vi "Alpha3.4.vi"() -> ()   [LabVIEW 2011]
uses:
  <vilib>/vision/NI_Vision_Development_Module.lvlib
panel:
  out "Image Enhanced":T1(plugin-control)
  in  "Kernel (Filters)":sgl[][](array[numeric])=array171x171[29241 elements]
  in  "Gray Morphology Operation":T2(ring)
  in  "Gamma":sgl(slide)=2.14 scale=0.0..10.0
  in  "Contrast":u8(slide)=60 scale=0.0..255.0
  in  "Brightness":u8(slide)=118 scale=0.0..255.0
  in  "Basic Morphology Operatoin":T3(ring)
  out "Contour Line":T1(plugin-control)
  in  "Threshold":cluster{u8, u8}(slide)={0, 6} scale=0.0..256.0
  in  "Stop":bool
  in  "Browse":bool
  out "Original Image":T1(plugin-control)
  out "Path to Image":path
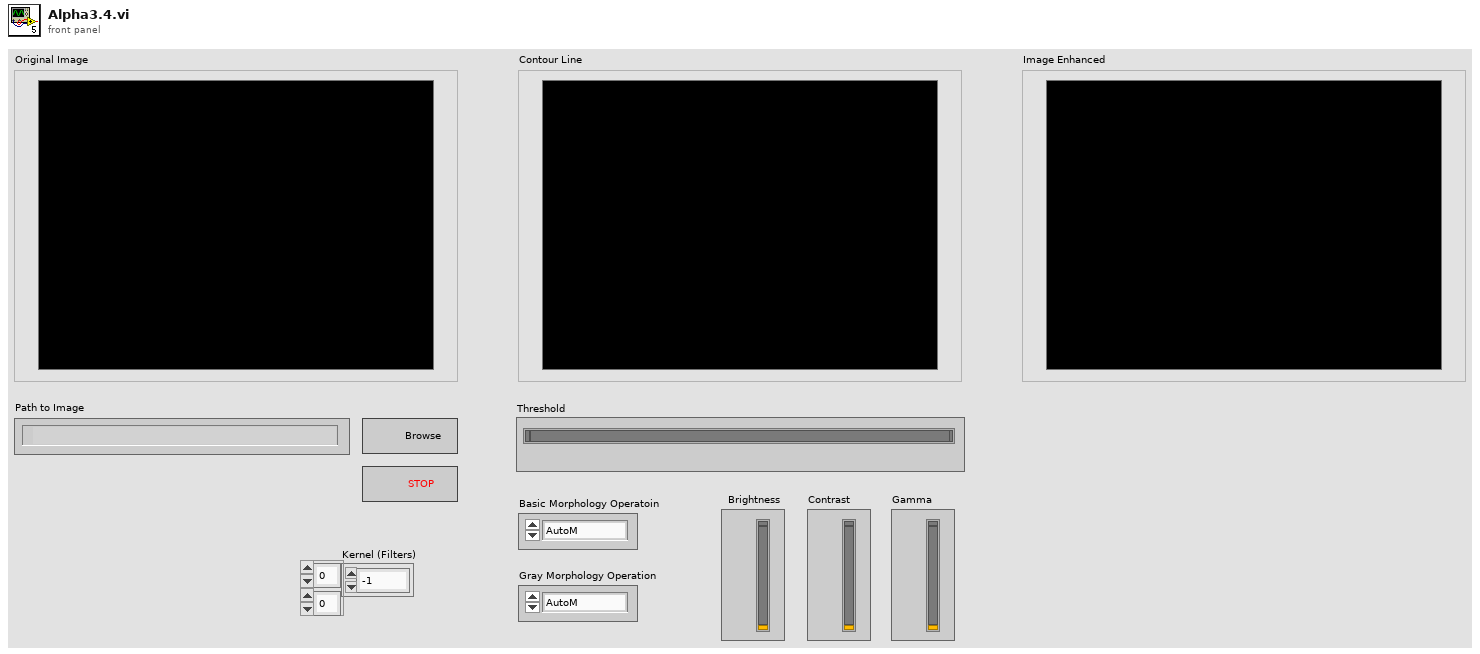
[diagram p1: front panel]
types:
  T1 = typedef "IMAQ Image.ctl" = refnum<image>
  T2 = enum16{"AutoM", "Close", "Dilate", "Erode", "Gradient", "Gradient in", "Gradient out", "HitMiss", "Open", "PClose", "POpen", "Thick", "Thin"}
  T3 = enum16{"AutoM", "Close", "Dilate", "Erode", "Gradient", "Gradient out", "Gradient in", "Hit miss", "Open", "PClose", "POpen", "Thick", "Thin"}
  T4 = typedef "Image Type" = u32
  T5 = cluster{"Brightness":u8, "Contrast":u8, "Gamma":sgl}
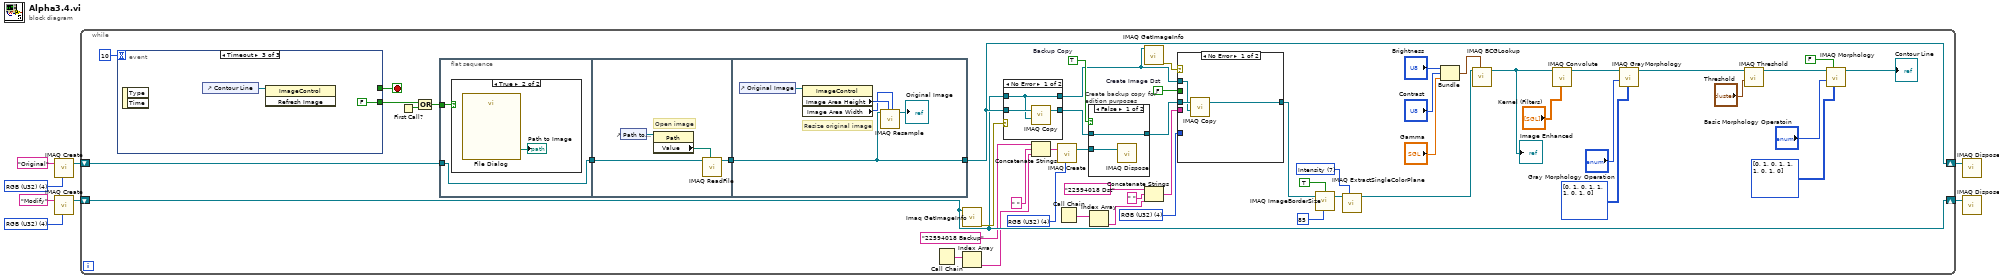
[diagram p0: block diagram]
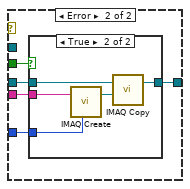
[diagram p2: hidden frame]
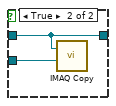
[diagram p4: hidden frame]
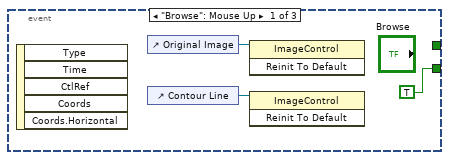
[diagram p7: hidden frame]
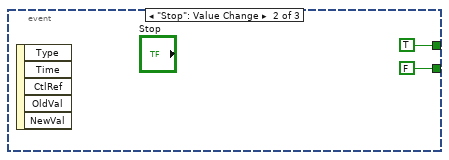
[diagram p8: hidden frame]
diagram:
  w1 = T4 4 items=["Grayscale (U8)", "Grayscale (I16)", "Grayscale (SGL)", "Complex (CSG)", "RGB (U32)", "HSL (U32)", "RGB (U64)", "Grayscale (U16)"] ("Image Type")
  w4 = T4 4 items=["Grayscale (U8)", "Grayscale (I16)", "Grayscale (SGL)", "Complex (CSG)", "RGB (U32)", "HSL (U32)", "RGB (U64)", "Grayscale (U16)"] ("Image Type")
  n1 = call "IMAQ Create"("Image Name"="Original", "Image Type"=w4) -> ("New Image"=w7:T1)  [unwired: 3 in, 1 out]
  n2 = call "IMAQ Create"("Image Name"="Modify", "Image Type"=w1) -> ("New Image"=w5:T1)  [unwired: 3 in, 1 out]
  n3 = while {
    shift-right: [w57] -> w3
    shift-left: w7 -> [w52]
    shift-right: [w56] -> w2
    shift-left: w5 -> [w56]
    stop <- w58 stop-if-true
    w38 = 7 items=["Red", "Green", "Blue", "Hue", "Saturation", "Luminance", "Value", "Intensity"] ("Color Plane")
    w34 = T4 4 items=["Grayscale (U8)", "Grayscale (I16)", "Grayscale (SGL)", "Complex (CSG)", "RGB (U32)", "HSL (U32)", "RGB (U64)", "Grayscale (U16)"] ("Image Dst Type")
    w33 = T4 4 items=["Grayscale (U8)", "Grayscale (I16)", "Grayscale (SGL)", "Complex (CSG)", "RGB (U32)", "HSL (U32)", "RGB (U64)", "Grayscale (U16)"] ("Image Type")
    w18 = TRUE  # Backup Copy
    w21 = FALSE  # Create Image Dst
    n4 = event shown="[2] Timeout" {
      selector: _ -> [_ _ _]
      dyn-events: _ -> [_ _ _]
      timeout: 10 -> [_ _ _]
      tunnel: [_ TRUE _] -> w58
      tunnel: [TRUE FALSE FALSE] -> w55
      event "Browse": Mouse Up {
        n5 = event-data() -> ()  [unwired: 1 in, 5 out]
        n6 = control-ref of="Original Image"() -> (w97:refnum<vi>)
        n7 = control-ref of="Contour Line"() -> (w98:refnum<vi>)
        n8 = invoke class="ImageControl" method="Reinit To Default"(reference=w97) -> ()  [unwired: 2 in, 3 out]
        n9 = invoke class="ImageControl" method="Reinit To Default"(reference=w98) -> ()  [unwired: 2 in, 3 out]
      }
      event "Stop": Value Change {
        n10 = event-data() -> ()  [unwired: 1 in, 5 out]
      }
      event Timeout {
        n11 = event-data() -> ()  [unwired: 1 in, 2 out]
        n12 = control-ref of="Contour Line"() -> (w102:refnum<vi>)
        n13 = invoke class="ImageControl" method="Refresh Image"(reference=w102) -> ()  [unwired: 2 in, 3 out]
      }
    }
    n14 = First Call?() -> (First Call?: T/F=w54:bool)
    n15 = Or(x=w55, y=w54) -> (x .or. y?=w53:bool)
    n16 = flat-sequence {
      tunnel: w53 -> [w85]
      tunnel: w52 -> [w84]
      tunnel: [w84] -> w51
      tunnel: [w90] -> w60
      tunnel: w51 -> [w87]
      tunnel: w60 -> [w91]
      tunnel: [w91] -> w57
      frame #0 {
        n17 = case shown="True" w85 {
          frame False {
          }
          frame True {
            n18 = call "File Dialog"() -> ("selected path"=→"Path to Image":path)  [unwired: 12 in, 3 out]
          }
        }
      }
      frame #1 {
        # "Open image"
        n19 = control-ref of="Path to Image"() -> (w89:refnum<vi>)
        n20 = property class="Path"(reference=w89) -> ("Value"=w88:path)  [unwired: 1 in, 2 out]
        n21 = call "IMAQ ReadFile"("File Path"=w88, "Image"=w87) -> ("Image Out"=w90:T1)  [unwired: 5 in, 4 out]
      }
      frame #2 {
        # "Resize original image"
        n22 = control-ref of="Original Image"() -> (w95:refnum<vi>)
        n23 = property class="ImageControl"(reference=w95) -> ("Image Area Height"=w94:u32, "Image Area Width"=w93:u32)  [unwired: 1 in, 2 out]
        n24 = call "IMAQ Resample"("X Resolution"=w93, "Y Resolution"=w94, "Image Src"=w91) -> ("Image Dst Out"=→"Original Image":T1)  [unwired: 7 in, 1 out]
      }
    }
    n25 = Call Chain() -> (call chain=w27:string[])
    n26 = call "Imaq GetImageInfo"("Image"=w56) -> ("error out"=w59:errorcluster)  [unwired: 1 in, 9 out]
    n27 = Index Array(array=w27) -> (element=w28:string)  [unwired: 1 in]
    n28 = case shown="No Error" w59 {
      tunnel: w56 -> [w80 w83]
      tunnel: w57 -> [w81 w82]
      tunnel: [w80 w83] -> w17
      tunnel: [w79 w82] -> w16
      frame No Error {
        n29 = call "IMAQ Copy"("Image Dst"=w80, "Image Src"=w81) -> ("Image Dst Out"=w79:T1)  [unwired: 4 in, 1 out]
      }
      frame Error {
      }
    }
    n30 = Concatenate Strings("22594018 Backup" ("Backup Image Name"), " ", w28) -> (w31:string)
    n31 = call "IMAQ Create"("Image Name"=w31, "Image Type"=w33) -> ("New Image"=w32:T1)  [unwired: 2 in, 2 out]
    n32 = Call Chain() -> (call chain=w22:string[])
    n33 = case "Create backup copy for edition purposes" shown="False" w18 {
      tunnel: [w76 w78] -> w20
      tunnel: w16 -> [w76 w78]
      tunnel: w32 -> [w75 w77]
      frame False {
        n34 = call "IMAQ Dispose"("Image"=w75) -> ()  [unwired: 2 in, 4 out]
      }
      frame True {
        n35 = call "IMAQ Copy"("Image Dst"=w77, "Image Src"=w78) -> ()  [unwired: 1 in, 5 out]
      }
    }
    n36 = Index Array(array=w22) -> (element=w24:string)  [unwired: 1 in]
    n37 = call "IMAQ GetImageInfo"("Image"=w17) -> ("error out"=w19:errorcluster)  [unwired: 1 in, 9 out]
    n38 = Concatenate Strings("22594018 Dst" ("Image Dst Name"), " ", w24) -> (w26:string)
    n39 = case shown="No Error" w19 {
      tunnel: [w63 w65] -> w35
      tunnel: w20 -> [w62 w66]
      tunnel: w17 -> [w61 _]
      tunnel: w26 -> [_ w68]
      tunnel: w34 -> [_ w67]
      tunnel: w21 -> [_ w64]
      frame No Error {
        n40 = call "IMAQ Copy"("Image Dst"=w61, "Image Src"=w62) -> ("Image Dst Out"=w63:T1)  [unwired: 1 in, 4 out]
      }
      frame Error {
        n41 = case shown="True" w64 {
          tunnel: w68 -> [_ w74]
          tunnel: w67 -> [_ w73]
          tunnel: w66 -> [w69 w71]
          tunnel: [w69 w70] -> w65
          frame False {
          }
          frame True {
            n42 = call "IMAQ Create"("Image Name"=w74, "Image Type"=w73) -> ("New Image"=w72:T1)  [unwired: 2 in, 2 out]
            n43 = call "IMAQ Copy"("Image Dst"=w72, "Image Src"=w71) -> ("Image Dst Out"=w70:T1)  [unwired: 1 in, 4 out]
          }
        }
      }
    }
    n44 = call "IMAQ ImageBorderSize"("Get/Set Status? (Set)"=TRUE, "Image"=w35, "Image border size in"=85 ("Border Size")) -> ("Image Out"=w39:T1)  [unwired: 1 in, 2 out]
    n45 = call "IMAQ ExtractSingleColorPlane"("Color Plane"=w38, "Image Src"=w39) -> ("Image Dst Out"=w40:T1)  [unwired: 2 in, 7 out]
    n46 = Bundle("Brightness"="Brightness", "Contrast"="Contrast", "Gamma"="Gamma") -> (w15:T5)  [unwired: 1 in]
    n47 = call "IMAQ BCGLookup"("Image Src"=w40, "BCG Values"=w15) -> ("Image Dst Out"=w9:T1)  [unwired: 3 in, 3 out]
    "Image Enhanced" <- w9
    n48 = call "IMAQ Convolute"("Kernel"="Kernel (Filters)", "Image Src"=w9) -> ("Image Dst Out"=w42:T1)  [unwired: 5 in, 4 out]
    n49 = call "IMAQ GrayMorphology"("Structuring Element"=i32[][] [[0, 1, 0], [1, 1, 1], [0, 1, 0]], "Operation"="Gray Morphology Operation", "Image Src"=w42) -> ("Image Dst Out"=w43:T1)  [unwired: 4 in, 4 out]
    n50 = call "IMAQ Threshold"("Range"="Threshold", "Image Src"=w43) -> ("Image Dst Out"=w46:T1)  [unwired: 4 in, 5 out]
    n51 = call "IMAQ Morphology"("Structuring Element"=i32[][] [[0, 1, 0], [1, 1, 1], [0, 1, 0]], "Square/Hexa (Square)"=FALSE, "Operation"="Basic Morphology Operatoin", "Image Src"=w46) -> ("Image Dst Out"=→"Contour Line":T1)  [unwired: 3 in, 4 out]
  }
  n52 = call "IMAQ Dispose"("Image"=w3) -> ()  [unwired: 5 in, 1 out]
  n53 = call "IMAQ Dispose"("Image"=w2) -> ()  [unwired: 5 in, 1 out]
